vi "serverG2.vi"() -> ()   [LabVIEW 2020]
panel:
  out "Charakterystyka":waveform(dbl)(graph)
  in  "stop 2":bool
  in  "Sygna³":T1(ring)
  in  "Amplituda":dbl(knob) scale=0.0..10.0
  in  "Czêstotliwoœæ":dbl(knob) scale=0.0..10.0
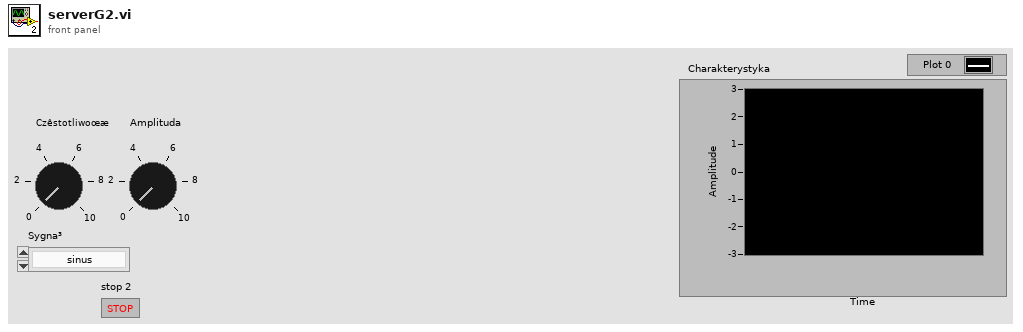
[diagram p1: front panel]
types:
  T1 = enum16{"sinus\n", "square\n", "triangle\n", "sawtooth\n"}
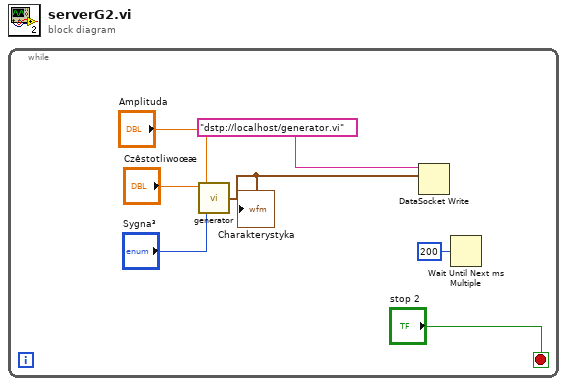
[diagram p0: block diagram]
diagram:
  n1 = while {
    stop <- "stop 2" stop-if-true
    n2 = call "generator.vi"("Sygna³"="Sygna³", "Amplituda"="Amplituda", "Czêstotliwoœæ"="Czêstotliwoœæ") -> ("Charakterystyka"=w3:waveform(dbl))  [unwired: 1 in]
    "Charakterystyka" <- w3
    n3 = DataSocket Write(10:w3, 11:"dstp://localhost/generator.vi" ("connection in")) -> ()  [unwired: 2 in, 3 out]
    n4 = Wait Until Next ms Multiple(millisecond multiple=u32 200) -> ()  [unwired: 1 out]
  }
